vi "Host-UART-State-Machine-Tester.vi"() -> ()   [LabVIEW 2017]
uses:
  <vilib>/FPGAPlugInAG/PXIe-6592R/niLvFpga_Open_PXIe-6592R.vi
  <vilib>/rvi/interface/common/dynamic/niFpgaDynamicAddResources.vi
  <vilib>/FPGAPlugInAG/Dynamic/niLvFpga_Download_Dynamic.vi
  <vilib>/Utility/error.llb/Error Cluster From Error Code.vi
  <vilib>/rvi/errors/niLvFpgaAdjustHostInterfaceError.vi
  <vilib>/FPGAPlugInAG/Dynamic/niLvFpga_Run_Dynamic.vi
  <vilib>/FPGAPlugInAG/Dynamic/niLvFpga_Close_Dynamic.vi
  <vilib>/rvi/interface/nirviOpenFPGA/nirviOpenFPGA.xnode
  FPGA Bitfiles/Fpga-Uart-State-Machine.lvbitx
  <vilib>/rvi/interface/nirviMethod/nirviMethod.xnode
  <vilib>/rvi/interface/nirviReadWriteControl/nirviReadWriteControl.xnode
  <vilib>/rvi/interface/nirviCloseFPGA/nirviCloseFPGA.xnode
  NiFpgaLv.dll
  <vilib>/rvi/interface/Simulation/niFpgaSimulationCallBeginRW.vi
  <vilib>/FPGAPlugInAG/Dynamic/niLvFpga_ReadFifo_Dynamic.vi
  <vilib>/rvi/errors/niLvFpgaMergeErrorWithErrorCode.vi
panel:
  out "DBG_PROBE_2":u64[](array[numeric])=[284773531510878, 72341272352779506, 72341276647747584, 72341280942715662, 72341285237683740, 72341289532651818, 72341293827619896, 72341298122587974, 72622777394266708, 144961812049167714, 284773531519502, 72341272352788130, 72341276647756208, 72341280942724286, 72341285237692364, 72341289532660442, 72341293827628520, 72341298122596598, 72622777394275332, 144961812049176338, 284773531528126, 72341272352796754, 72341276647764832, 72341280942732910, 72341285237700988, 72341289532669066, 72341293827637144, 72341298122605222, 72622777394283956, 144961812049184962, 284773531536750, 72341272352805378, 72341276647773456, 72341280942741534, 72341285237709612, 72341289532677690, 72341293827645768, 72341298122613846, 72622777394292580, 144961812049193586, 284773531545374, 72341272352814002, 72341276647782080, 72341280942750158, 72341285237718236, 72341289532686314, 72341293827654392, 72341298122622470, 72622777394301204, 144961812049202210, 284773531553998, 72341272352822626, 72341276647790704, 72341280942758782, 72341285237726860, 72341289532694938, 72341293827663016, 72341298122631094, 72622777394309828, 144961812049210834, 284773531562622, 72341272352831250, 72341276647799328, 72341280942767406, 72341285237735484, 72341289532703562, 72341293827671640, 72341298122639718, 72622777394318452, 144961812049219458, 284773531571246, 72341272352839874, 72341276647807952, 72341280942776030, 72341285237744108, 72341289532712186, 72341293827680264, 72341298122648342, 72622777394327076, 144961812049228082, 284773531579870, 72341272352848498, 72341276647816576, 72341280942784654, 72341285237752732, 72341289532720810, 72341293827688888, 72341298122656966, 72622777394335700, 144961812049236706, 284773531588494, 72341272352857122, 72341276647825200, 72341280942793278, 72341285237761356, 72341289532729434, 72341293827697512, 72341298122665590, 72622777394344324, 144961812049245330, 284773531597118, 72341272352865746, 72341276647833824, 72341280942801902, 72341285237769980, 72341289532738058, 72341293827706136, 72341298122674214, 72622777394352948, 144961812049253954, 284773531605742, 72341272352874370, 72341276647842448, 72341280942810526, 72341285237778604, 72341289532746682, 72341293827714760, 72341298122682838, 72622777394361572, 144961812049262578, 284773531614366, 72341272352882994, 72341276647851072, 72341280942819150, 72341285237787228, 72341289532755306, 72341293827723384, 72341298122691462, 72622777394370196, 144961812049271202, 284773531622990, 72341272352891618, 72341276647859696, 72341280942827774, 72341285237795852, 72341289532763930, 72341293827732008, 72341298122700086, 72622777394378820, 144961812049279826, 284773531631614, 72341272352900242, 72341276647868320, 72341280942836398, 72341285237804476, 72341289532772554, 72341293827740632, 72341298122708710, 72622777394387444, 144961812049288450, 284773531640238, 72341272352908866, 72341276647876944, 72341280942845022, 72341285237813100, 72341289532781178, 72341293827749256, 72341298122717334, 72622777394396068, 144961812049297074, 284773531648862, 72341272352917490, 72341276647885568, 72341280942853646, 72341285237821724, 72341289532789802, 72341293827757880, 72341298122725958, 72622777394404692, 144961812049305698, 284773531657486, 72341272352926114, 72341276647894192, 72341280942862270, 72341285237830348, 72341289532798426, 72341293827766504, 72341298122734582, 72622777394413316, 144961812049314322, 284773531666110, 72341272352934738, 72341276647902816, 72341280942870894, 72341285237838972, 72341289532807050, 72341293827775128, 72341298122743206, 72622777394421940, 144961812049322946, 284773531674734, 72341272352943362, 72341276647911440, 72341280942879518, 72341285237847596, 72341289532815674, 72341293827783752, 72341298122751830, 72622777394430564, 144961812049331570, 284773531683358, 72341272352951986, 72341276647920064, 72341280942888142, 72341285237856220, 72341289532824298, 72341293827792376, 72341298122760454, 72622777394439188, 144961812049340194, 284773531691982, 72341272352960610, 72341276647928688, 72341280942896766, 72341285237864844, 72341289532832922, 72341293827801000, 72341298122769078, 72622777394447812, 144961812049348818, 284773531700606, 72341272352969234, 72341276647937312, 72341280942905390, 72341285237873468, 72341289532841546, 72341293827809624, 72341298122777702, 72622777394456436, 144961812049357442, 284773531709230, 72341272352977858, 72341276647945936, 72341280942914014, 72341285237882092, 72341289532850170, 72341293827818248, 72341298122786326, 72622777394465060, 144961812049366066, 284773531717854, 72341272352986482, 72341276647954560, 72341280942922638, 72341285237890716, 72341289532858794, 72341293827826872, 72341298122794950, 72622777394473684, 144961812049374690, 284773531726478, 72341272352995106, 72341276647963184, 72341280942931262, 72341285237899340, 72341289532867418, 72341293827835496, 72341298122803574, 72622777394482308, 144961812049383314, 284773531735102, 72341272353003730, 72341276647971808, 72341280942939886, 72341285237907964, 72341289532876042, 72341293827844120, 72341298122812198, 72622777394490932, 144961812049391938, 284773531743726, 72341272353012354, 72341276647980432, 72341280942948510, 72341285237916588, 72341289532884666, 72341293827852744, 72341298122820822, 72622777394499556, 144961812049400562, 284773531752350, 72341272353020978, 72341276647989056, 72341280942957134, 72341285237925212, 72341289532893290, 72341293827861368, 72341298122829446, 72622777394508180, 144961812049409186, 284773531760974, 72341272353029602, 72341276647997680, 72341280942965758, 72341285237933836, 72341289532901914, 72341293827869992, 72341298122838070, 72622777394516804, 144961812049417810, 284773531769598, 72341272353038226, 72341276648006304, 72341280942974382, 72341285237942460, 72341289532910538, 72341293827878616, 72341298122846694, 72622777394525428, 144961812049426434, 284773531778222, 72341272353046850, 72341276648014928, 72341280942983006, 72341285237951084, 72341289532919162, 72341293827887240, 72341298122855318, 72622777394534052, 144961812049435058, 284773531786846, 72341272353055474, 72341276648023552, 72341280942991630, 72341285237959708, 72341289532927786, 72341293827895864, 72341298122863942, 72622777394542676, 144961812049443682, 284773531795470, 72341272353064098, 72341276648032176, 72341280943000254, 72341285237968332, 72341289532936410, 72341293827904488, 72341298122872566, 72622777394551300, 144961812049452306, 284773531804094, 72341272353072722, 72341276648040800, 72341280943008878, 72341285237976956, 72341289532945034, 72341293827913112, 72341298122881190, 72622777394559924, 144961812049460930, 284773531812718, 72341272353081346, 72341276648049424, 72341280943017502, 72341285237985580, 72341289532953658, 72341293827921736, 72341298122889814, 72622777394568548, 144961812049469554, 284773531821342, 72341272353089970, 72341276648058048, 72341280943026126, 72341285237994204, 72341289532962282, 72341293827930360, 72341298122898438, 72622777394577172, 144961812049478178, 284773531829966, 72341272353098594, 72341276648066672, 72341280943034750, 72341285238002828, 72341289532970906, 72341293827938984, 72341298122907062, 72622777394585796, 144961812049486802, 284773531838590, 72341272353107218, 72341276648075296, 72341280943043374, 72341285238011452, 72341289532979530, 72341293827947608, 72341298122915686, 72622777394594420, 144961812049495426, 284773531847214, 72341272353115842, 72341276648083920, 72341280943051998, 72341285238020076, 72341289532988154, 72341293827956232, 72341298122924310, 72622777394603044, 144961812049504050, 284773531855838, 72341272353124466, 72341276648092544, 72341280943060622, 72341285238028700, 72341289532996778, 72341293827964856, 72341298122932934, 72622777394611668, 144961812049512674, 284773531864462, 72341272353133090, 72341276648101168, 72341280943069246, 72341285238037324, 72341289533005402, 72341293827973480, 72341298122941558, 72622777394620292, 144961812049521298, 284773531873086, 72341272353141714, 72341276648109792, 72341280943077870, 72341285238045948, 72341289533014026, 72341293827982104, 72341298122950182, 72622777394628916, 144961812049529922, 284773531881710, 72341272353150338, 72341276648118416, 72341280943086494, 72341285238054572, 72341289533022650, 72341293827990728, 72341298122958806, 72622777394637540, 144961812049538546, 284773531890334, 72341272353158962, 72341276648127040, 72341280943095118, 72341285238063196, 72341289533031274, 72341293827999352, 72341298122967430, 72622777394646164, 144961812049547170, 284773531898958, 72341272353167586, 72341276648135664, 72341280943103742, 72341285238071820, 72341289533039898, 72341293828007976, 72341298122976054, 72622777394654788, 144961812049555794, 284773531907582, 72341272353176210, 72341276648144288, 72341280943112366, 72341285238080444, 72341289533048522, 72341293828016600, 72341298122984678, 72622777394663412, 144961812049564418, 284773531916206, 72341272353184834, 72341276648152912, 72341280943120990, 72341285238089068, 72341289533057146, 72341293828025224, 72341298122993302, 72622777394672036, 144961812049573042, 284773531924830, 72341272353193458, 72341276648161536, 72341280943129614, 72341285238097692, 72341289533065770, 72341293828033848, 72341298123001926, 72622777394680660, 144961812049581666, 284773531933454, 72341272353202082, 72341276648170160, 72341280943138238, 72341285238106316, 72341289533074394, 72341293828042472, 72341298123010550, 72622777394689284, 144961812049590290, 284773531942078, 72341272353210706, 72341276648178784, 72341280943146862, 72341285238114940, 72341289533083018, 72341293828051096, 72341298123019174, 72622777394697908, 144961812049598914, 284773531950702, 72341272353219330, 72341276648187408, 72341280943155486, 72341285238123564, 72341289533091642, 72341293828059720, 72341298123027798, 72622777394706532, 144961812049607538, 284773531959326, 72341272353227954, 72341276648196032, 72341280943164110, 72341285238132188, 72341289533100266, 72341293828068344, 72341298123036422, 72622777394715156, 144961812049616162, 284773531967950, 72341272353236578, 72341276648204656, 72341280943172734, 72341285238140812, 72341289533108890, 72341293828076968, 72341298123045046, 72622777394723780, 144961812049624786, 284773531976574, 72341272353245202, 72341276648213280, 72341280943181358, 72341285238149436, 72341289533117514, 72341293828085592, 72341298123053670, 72622777394732404, 144961812049633410, 284773531985198, 72341272353253826, 72341276648221904, 72341280943189982, 72341285238158060, 72341289533126138, 72341293828094216, 72341298123062294, 72622777394741028, 144961812049642034, 284773531993822, 72341272353262450, 72341276648230528, 72341280943198606, 72341285238166684, 72341289533134762, 72341293828102840, 72341298123070918, 72622777394749652, 144961812049650658, 284773532002446, 72341272353271074, 72341276648239152, 72341280943207230, 72341285238175308, 72341289533143386, 72341293828111464, 72341298123079542, 72622777394758276, 144961812049659282] format="%.0x"
  out "DBG_PROBE_3":u64[](array[numeric])=[0, 0, 0, 0, 16777480, 264, 264, 16777800, 584, 584, 0, 16777473, 257, 16777733, 517, 517, 16778021, 16778341, 1125, 1125, 0, 0, 0, 16777476, 16777740, 524, 16778028, 16778348, 1132, 1132, 0, 0, 0, 16777476, 16777740, 524, 16778028, 16778348, 1132, 1132, 0, 16777473, 16777731, 16777991, 16778255, 1039, 16778543, 16778863, 1647, 1647, 0, 0, 0, 0, 0, 0, 16777504, 288, 288, 16777504, 0, 16777473, 16777731, 16777991, 775, 16778263, 1047, 16778583, 1367, 16778583, 0, 16777473, 16777731, 16777991, 16778255, 1039, 16778543, 16778863, 1647, 1647, 0, 0, 16777474, 258, 258, 16777746, 16778034, 16778354, 1138, 1138, 0, 0, 0, 16777476, 16777740, 524, 16778028, 16778348, 1132, 1132, 0, 0, 0, 16777476, 260, 260, 16777764, 16778084, 868, 16778084, 0, 0, 0, 0, 0, 0, 16777504, 288, 288, 16777504, 0, 0, 16777474, 16777734, 518, 518, 16778022, 16778342, 1126, 1126, 0, 0, 16777474, 258, 258, 16777746, 16778034, 16778354, 1138, 1138, 0, 16777473, 16777731, 16777991, 16778255, 1039, 16778543, 16778863, 1647, 1647, 0, 16777473, 257, 16777733, 16777997, 781, 16778285, 16778605, 1389, 16778605, 0, 0, 0, 0, 0, 0, 16777504, 288, 288, 16777504, 0, 16777473, 257, 16777733, 517, 16778005, 789, 16778325, 1109, 1109, 0, 16777473, 257, 257, 257, 257, 257, 16777793, 577, 577, 0, 0, 16777474, 258, 258, 16777746, 530, 16778066, 850, 16778066, 0, 0, 0, 16777476, 260, 16777748, 532, 16778068, 852, 16778068, 0, 0, 0, 0, 0, 0, 16777504, 288, 288, 16777504, 0, 0, 0, 16777476, 260, 16777748, 532, 16778068, 852, 16778068, 0, 16777473, 257, 16777733, 517, 517, 16778021, 16778341, 1125, 1125, 0, 16777473, 16777731, 515, 515, 16778003, 16778291, 16778611, 1395, 16778611, 0, 0, 0, 16777476, 260, 16777748, 16778036, 16778356, 1140, 1140, 0, 16777473, 257, 257, 257, 257, 16777761, 545, 545, 545, 0, 16777473, 257, 16777733, 16777997, 781, 781, 781, 781, 16777997, 0, 0, 16777474, 258, 16777738, 522, 522, 522, 522, 522, 0, 16777473, 16777731, 16777991, 16778255, 1039, 1039, 16778575, 1359, 16778575, 0, 0, 0, 16777476, 16777740, 524, 16778028, 16778348, 1132, 1132, 0, 0, 0, 16777476, 260, 260, 16777764, 16778084, 868, 16778084, 0, 0, 0, 0, 0, 0, 16777504, 288, 288, 16777504, 0, 0, 16777474, 16777734, 518, 16778006, 790, 16778326, 1110, 1110, 0, 16777473, 257, 257, 257, 257, 16777761, 16778081, 865, 16778081, 0, 0, 0, 16777476, 16777740, 524, 16778028, 16778348, 1132, 1132, 0, 16777473, 257, 16777733, 517, 16778005, 16778293, 16778613, 1397, 16778613, 0, 16777473, 257, 16777733, 517, 517, 16778021, 16778341, 1125, 1125, 0, 0, 16777474, 258, 16777738, 16778010, 16778298, 1082, 1082, 1082, 0, 0, 0, 0, 0, 0, 16777504, 288, 288, 16777504, 0, 0, 0, 0, 0, 16777488, 16777776, 560, 560, 560, 0, 0, 0, 16777476, 16777740, 524, 16778028, 812, 812, 16778028, 0, 0, 0, 0, 0, 0, 16777504, 288, 288, 16777504, 0, 0, 16777474, 16777734, 16777998, 782, 782, 16778318, 1102, 1102, 0, 16777473, 257, 16777733, 517, 517, 16778021, 16778341, 1125, 1125, 0, 16777473, 16777731, 16777991, 775, 16778263, 16778551, 16778871, 1655, 1655, 0, 0, 0, 0, 0, 0, 16777504, 288, 288, 16777504, 0, 0, 16777474, 16777734, 518, 16778006, 790, 16778326, 1110, 1110, 0, 16777473, 257, 257, 257, 257, 16777761, 16778081, 865, 16778081, 0, 0, 0, 16777476, 16777740, 524, 16778028, 16778348, 1132, 1132, 0, 16777473, 257, 16777733, 517, 16778005, 16778293, 16778613, 1397, 16778613, 0, 16777473, 257, 16777733, 517, 517, 16778021, 16778341, 1125, 1125, 0, 0, 16777474, 258, 16777738, 16778010, 16778298, 1082, 1082, 1082, 0, 0, 0, 0, 0, 0, 16777504, 288, 288, 16777504, 0, 16777473, 16777731, 16777991, 775, 16778263, 16778551, 1335, 1335, 16778551, 0, 16777473, 257, 16777733, 16777997, 781, 781, 781, 781, 16777997, 0, 16777473, 257, 16777733, 16777997, 781, 781, 781, 781, 16777997, 0, 0, 16777474, 258, 16777738, 522, 522, 522, 522, 522] format="%.0x"
  in  "reset_rtl":bool=TRUE
  out "DBG_PROBE":u64[](array[numeric])=[19916894, 4314887327, 19920815, 4314889679, 19923167, 4314892030, 19925518, 4314893599, 19927087, 4314895167, 19928655, 4314897519, 19931791, 4314900654, 19934142, 4314903791, 19938063, 4314906143, 19940415, 4314909278, 19942766, 4314912415, 19946687, 4314914767, 19949039, 4314917902, 19951390, 4314919471, 19955311, 4314923391, 19957663, 4314926526, 19960014, 4314932015, 19965503, 4314934367, 19968638, 4314936719, 19971775, 4314939855, 19973343, 4314941423, 19974911, 4314942991, 19977262, 4314945343, 19981183, 4314949263, 19983535, 4314952398, 19985886, 4314954751, 19988239, 4314957103, 19992159, 4314961022, 19994510, 4314964159, 19998431, 4314966511, 20000783, 4314969646, 20003134, 4314972783, 20006271, 4314975135, 20009407, 4314977487, 20011758, 4314983759, 20017247, 4314986111, 20020382, 4314989247, 20023519, 4314992383, 20026655, 4314995518, 20029006, 4314997871, 20031359, 4315000223, 20035279, 4315004142, 20037630, 4315005711, 20041551, 4315009631, 20043903, 4315012766, 20046254, 4315014335, 20047823, 4315015903, 20050175, 4315018255, 20052527, 4315020607, 20054878, 4315026879, 20060367, 4315029231, 20063502, 4315031583, 20065071, 4315033151, 20066639, 4315034719, 20068207, 4315036287, 20069775, 4315038638, 20072126, 4315040207, 20073695, 4315044911, 20078399, 4315047262, 20080750, 4315049615, 20083103, 4315051967, 20085455, 4315053535, 20087023, 4315055103, 20089374, 4315059023, 20092511, 4315060591, 20094079, 4315062159, 20095647, 4315063727, 20097998, 4315069999, 20103487, 4315072351, 20106622, 4315076271, 20109759, 4315077839, 20111327, 4315079407, 20112895, 4315080975, 20115246, 4315083327, 20116815, 4315084895, 20118383, 4315087247, 20121519, 4315090382, 20123870, 4315091951, 20126223, 4315095087, 20130143, 4315098223, 20132494, 4315102143, 20135631, 4315103711, 20138767, 4315107630, 20141118, 4315109199, 20142687, 4315113119, 20146607, 4315116254, 20149742, 4315117823, 20151311, 4315119391, 20153663, 4315124095, 20158366, 4315127231, 20160719, 4315128799, 20162287, 4315133502, 20166990, 4315135071, 20170911, 4315139775, 20173263, 4315141343, 20175614, 4315145263, 20179535, 4315147615, 20181887, 4315150750, 20184238, 4315153887, 20187375, 4315156239, 20190511, 4315158591, 20192862, 4315164863, 20198351, 4315167215, 20201486, 4315170351, 20204623, 4315172703, 20206191, 4315174271, 20207759, 4315176622, 20210110, 4315178191, 20211679, 4315182111, 20216383, 4315184463, 20218734, 4315188383, 20222655, 4315190735, 20225007, 4315193870, 20227358, 4315195439, 20228927, 4315197007, 20230495, 4315198575, 20233631, 4315201711, 20235982, 4315204063, 20237551, 4315205631, 20239119, 4315207983, 20242255, 4315211118, 20244606, 4315213471, 20246959, 4315215039, 20250095, 4315219742, 20253230, 4315225231, 20258719, 4315227583, 20261854, 4315233071, 20267343, 4315236990, 20270478, 4315240127, 20274399, 4315242479, 20275967, 4315244831, 20279102, 4315251103, 20284591, 4315253455, 20287726, 4315256591, 20291647, 4315260511, 20293999, 4315262862, 20296350, 4315264431, 20297919, 4315265999, 20299487, 4315268351, 20302623, 4315271486, 20304974, 4315273055, 20308111, 4315276191, 20311247, 4315280110, 20313598, 4315285599, 20319087, 4315287951, 20322222, 4315291087, 20325359, 4315293439, 20326927, 4315295007, 20328495, 4315297358, 20330846, 4315298927, 20332415, 4315302847, 20337119, 4315305199, 20339470, 4315309119, 20343391, 4315311471, 20345743, 4315314606, 20348094, 4315316175, 20349663, 4315317743, 20351231, 4315319311, 20354367, 4315322447, 20356718, 4315324799, 20358287, 4315326367, 20359855, 4315328719, 20362991, 4315331854, 20365342, 4315334207, 20367695, 4315335775, 20370831, 4315340478, 20373966, 4315345967, 20379455, 4315348319, 20382590, 4315350671, 20385727, 4315353807, 20388079, 4315356943, 20391214, 4315359295, 20392783, 4315360863, 20395135, 4315365567, 20399838, 4315367919, 20401407, 4315369487, 20403759, 4315374191, 20408462, 4315377327, 20410815, 4315378895, 20412383, 4315383598] format="%.0x"
  in  "d_microblaze_i\\uart_rtl_rxd":bool=TRUE
  out "gpio_rtl_0_tri_o":u32=771 format="%.0x"
  in  "gpio_rtl_tri_i":u32=7
  out "Baud Rate 2":u32=128000
  out "error out":errorcluster
  out "UART Data":u8[](array[numeric])=[72, 101, 108, 108, 111, 32, 87, 111, 114, 108, 100, 32, 102, 114, 111, 109, 32, 85, 65, 82, 84, 32, 84, 101, 115, 116, 33, 13, 10, 79, 108, 100, 32, 86, 97, 108, 117, 101, 58, 32, 48, 44, 32, 78, 101, 119, 32, 86, 97, 108, 117, 101, 58, 32, 55, 13, 13, 10] format="%.0x"
  in  "stop":bool
  in  "FPGA Clock Rate (MHz)":u32=100
  in  "Baud Rate":u32=128000
  in  "error in":errorcluster
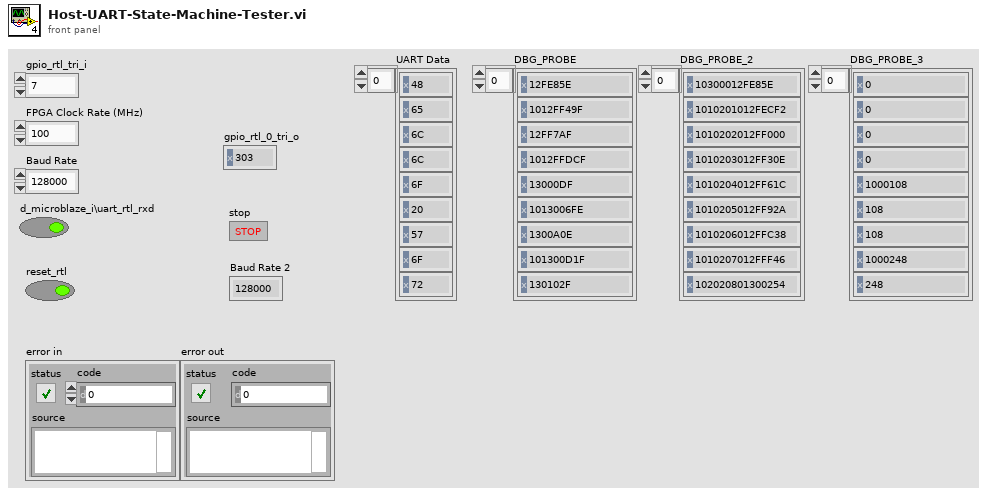
[diagram p1: front panel]
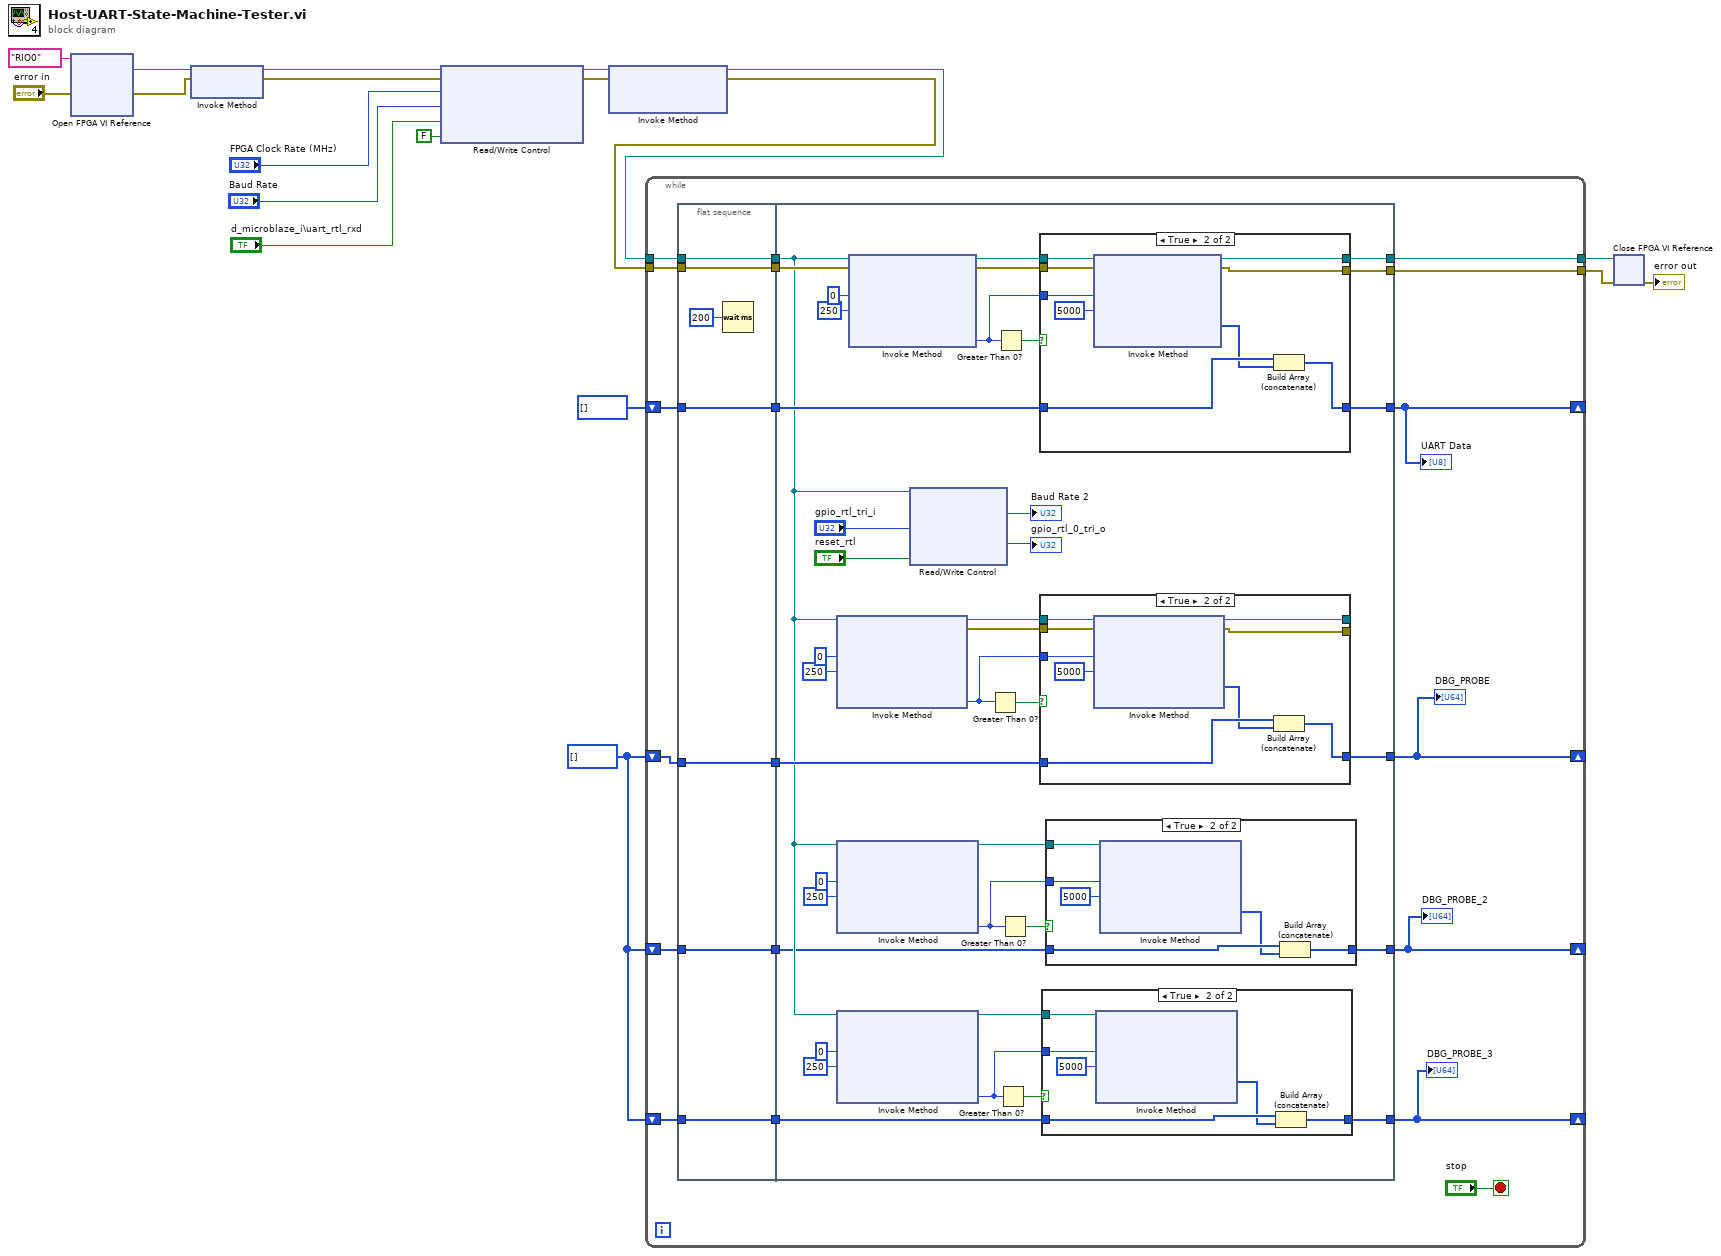
[diagram p0: block diagram]
diagram:
  w2 = u64[] []
  n1 = xnode "Open FPGA VI Reference"("error in"="error in", "resource name"=tag "RIO0") -> ("FPGA VI Reference Out"=w18:refnum<k20>, "error out"=w4:errorcluster)
  n2 = xnode "Invoke Method"("FPGA VI Reference In"=w18, "error in"=w4) -> ("FPGA VI Reference Out"=w5:refnum<k20>, "error out"=w3:errorcluster)
  n3 = xnode "Read/Write Control"("FPGA VI Reference In"=w5, "error in"=w3, "FPGA Clock Rate (MHz)"="FPGA Clock Rate (MHz)", "Baud Rate"="Baud Rate", "uart_rtl_rxd"="d_microblaze_i\\uart_rtl_rxd", "reset_rtl"=FALSE) -> ("FPGA VI Reference Out"=w15:refnum<k20>, "error out"=w14:errorcluster)
  n4 = xnode "Invoke Method"("FPGA VI Reference In"=w15, "error in"=w14) -> ("FPGA VI Reference Out"=w13:refnum<k20>, "error out"=w12:errorcluster)  [unwired: 1 in]
  n5 = while {
    tunnel: w13 -> [w36]
    tunnel: w12 -> [w35]
    shift-right: [w31] -> _
    shift-left: u8[] [] -> [w33]
    tunnel: [w30] -> w10
    tunnel: [w29] -> w9
    shift-right: [w26] -> _
    shift-left: w2 -> [w28]
    shift-right: [w20] -> _
    shift-left: w2 -> [w24]
    shift-right: [w21] -> _
    shift-left: w2 -> [w23]
    stop <- "stop" stop-if-true
    n6 = flat-sequence {
      tunnel: [w44] -> w38
      tunnel: w36 -> [w44]
      tunnel: [w43] -> w37
      tunnel: w35 -> [w43]
      tunnel: w33 -> [w42]
      tunnel: [w42] -> w32
      tunnel: w28 -> [w41]
      tunnel: [w41] -> w27
      tunnel: [w40] -> w25
      tunnel: w24 -> [w40]
      tunnel: w23 -> [w39]
      tunnel: [w39] -> w22
      tunnel: w38 -> [w56]
      tunnel: w37 -> [w83]
      tunnel: w32 -> [w76]
      tunnel: [w75] -> w31
      tunnel: [w74] -> w30
      tunnel: [w73] -> w29
      tunnel: w27 -> [w67]
      tunnel: [w64] -> w26
      tunnel: w25 -> [w53]
      tunnel: [w52] -> w20
      tunnel: w22 -> [w50]
      tunnel: [w48] -> w21
      frame #0 {
        n7 = Wait (ms)(milliseconds to wait=u32 200) -> ()  [unwired: 1 out]
      }
      frame #1 {
        n8 = xnode "Invoke Method"("FPGA VI Reference In"=w56, "Number of Elements"=u32 0, "Timeout (ms)"=250) -> ("FPGA VI Reference Out"=w69:refnum<k20>, "error out"=w68:errorcluster, "Elements Remaining"=w65:u32)  [unwired: 1 in, 1 out]
        n9 = xnode "Invoke Method"("FPGA VI Reference In"=w56, "Number of Elements"=u32 0, "Timeout (ms)"=250) -> ("FPGA VI Reference Out"=w55:refnum<k20>, "Elements Remaining"=w51:u32)  [unwired: 1 in, 2 out]
        n10 = xnode "Invoke Method"("FPGA VI Reference In"=w56, "Number of Elements"=u32 0, "Timeout (ms)"=250) -> ("FPGA VI Reference Out"=w49:refnum<k20>, "Elements Remaining"=w46:u32)  [unwired: 1 in, 2 out]
        n11 = xnode "Invoke Method"("FPGA VI Reference In"=w56, "error in"=w83, "Number of Elements"=u32 0, "Timeout (ms)"=250) -> ("FPGA VI Reference Out"=w79:refnum<k20>, "error out"=w78:errorcluster, "Elements Remaining"=w77:u32)  [unwired: 1 out]
        n12 = xnode "Read/Write Control"("FPGA VI Reference In"=w56, "gpio_rtl_tri_i"="gpio_rtl_tri_i", "reset_rtl"="reset_rtl") -> ("Baud Rate"=→"Baud Rate 2":u32, "gpio_rtl_0_tri_o"=→"gpio_rtl_0_tri_o":u32)  [unwired: 1 in, 2 out]
        n13 = Greater Than 0?(x=w65) -> (x > 0?=w66:bool)
        n14 = Greater Than 0?(x=w77) -> (x > 0?=w80:bool)
        n15 = Greater Than 0?(x=w46) -> (x > 0?=w47:bool)
        n16 = Greater Than 0?(x=w51) -> (x > 0?=w54:bool)
        n17 = case shown="True" w80 {
          tunnel: w79 -> [w110 w121]
          tunnel: w78 -> [w111 w120]
          tunnel: w77 -> [_ w119]
          tunnel: w76 -> [w112 w117]
          tunnel: [w112 w115] -> w75
          tunnel: [w110 w114] -> w74
          tunnel: [w111 w113] -> w73
          frame False {
          }
          frame True {
            n18 = xnode "Invoke Method"("FPGA VI Reference In"=w121, "error in"=w120, "Number of Elements"=w119, "Timeout (ms)"=5000) -> ("FPGA VI Reference Out"=w114:refnum<k20>, "error out"=w113:errorcluster, "Data"=w116:u8[])  [unwired: 1 out]
            n19 = Build Array (concatenate)(w117, w116) -> (w115:u8[])
          }
        }
        n20 = case shown="True" w66 {
          tunnel: w69 -> [w98 w109]
          tunnel: w68 -> [w99 w108]
          tunnel: w65 -> [_ w107]
          tunnel: w67 -> [w100 w105]
          tunnel: [w100 w103] -> w64
          tunnel: [w98 w102] -> _
          tunnel: [w99 w101] -> _
          frame False {
          }
          frame True {
            n21 = xnode "Invoke Method"("FPGA VI Reference In"=w109, "error in"=w108, "Number of Elements"=w107, "Timeout (ms)"=5000) -> ("FPGA VI Reference Out"=w102:refnum<k20>, "error out"=w101:errorcluster, "Data"=w104:u64[])  [unwired: 1 out]
            n22 = Build Array (concatenate)(w105, w104) -> (w103:u64[])
          }
        }
        n23 = case shown="True" w47 {
          tunnel: w49 -> [_ w90]
          tunnel: w46 -> [_ w89]
          tunnel: w50 -> [w84 w87]
          tunnel: [w84 w85] -> w48
          frame False {
          }
          frame True {
            n24 = xnode "Invoke Method"("FPGA VI Reference In"=w90, "Number of Elements"=w89, "Timeout (ms)"=5000) -> ("Data"=w86:u64[])  [unwired: 1 in, 3 out]
            n25 = Build Array (concatenate)(w87, w86) -> (w85:u64[])
          }
        }
        n26 = case shown="True" w54 {
          tunnel: w55 -> [_ w97]
          tunnel: w51 -> [_ w96]
          tunnel: w53 -> [w91 w94]
          tunnel: [w91 w92] -> w52
          frame False {
          }
          frame True {
            n27 = xnode "Invoke Method"("FPGA VI Reference In"=w97, "Number of Elements"=w96, "Timeout (ms)"=5000) -> ("Data"=w93:u64[])  [unwired: 1 in, 3 out]
            n28 = Build Array (concatenate)(w94, w93) -> (w92:u64[])
          }
        }
      }
    }
    "UART Data" <- w31
    "DBG_PROBE" <- w26
    "DBG_PROBE_3" <- w21
    "DBG_PROBE_2" <- w20
  }
  n29 = xnode "Close FPGA VI Reference"("FPGA VI Reference In"=w10, "error in"=w9) -> ("error out"=→"error out":errorcluster)
